vi "DCA Convert Measurement Cluster.vi"(4 "Conversion":enum16{"Cluster - HTML", "HTML - Cluster"}(ring), 6 "Measurements Key Array In":T4, 7 "Measurements Cluster In":T1={"Topology"=enum."PI-Network", "Lock Topology"=FALSE, "ATTN Calc"=enum."Power", "Zo"=50.0}) -> (1 "Measurements Cluster Out":T1={"Topology"=enum."PI-Network", "Lock Topology"=FALSE, "ATTN Calc"=enum."Power", "Zo"=50.0}, 2 "Measurements HTML Out":string)   [LabVIEW 2011]
uses:
  Addons/internet/utils/keyedarr.llb/Keyed Array.ctl
  TypeDefs/DCA Measurement Cluster.ctl
  TypeDefs/DCA Topology.ctl
  TypeDefs/DCA Attenuation Calculation.ctl
  Addons/internet/utils/strutil.llb/Case Matching.ctl
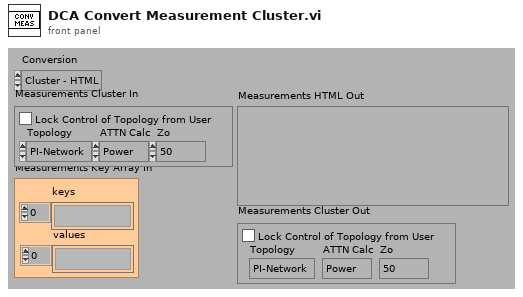
[diagram p1: front panel]
types:
  T1 = typedef "DCA Measurement Cluster.ctl" = cluster{"Topology":T2, "Lock Topology":bool, "ATTN Calc":T3, "Zo":dbl}
  T2 = typedef "DCA Topology.ctl" = enum32{"PI-Network", "T-Network"}
  T3 = typedef "DCA Attenuation Calculation.ctl" = enum32{"Power", "Voltage"}
  T4 = typedef "Keyed Array.ctl" = cluster{"keys":string[], "values":string[]}
  T5 = typedef "Case Matching.ctl" = enum16{"a != A", "a == A", "system"}
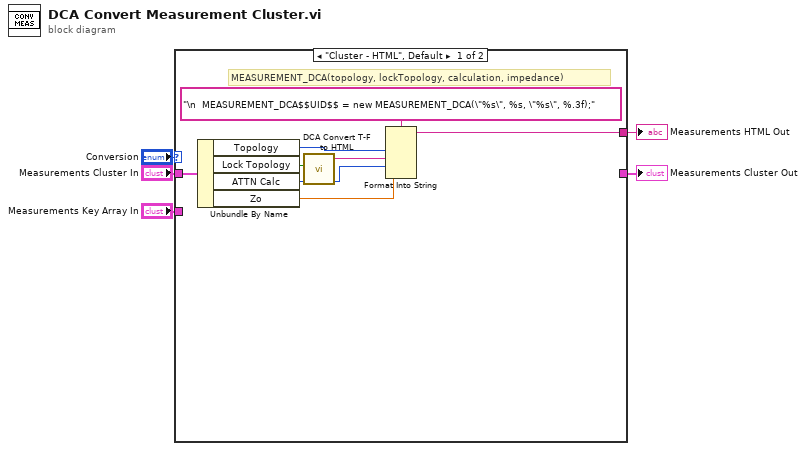
[diagram p0: block diagram]
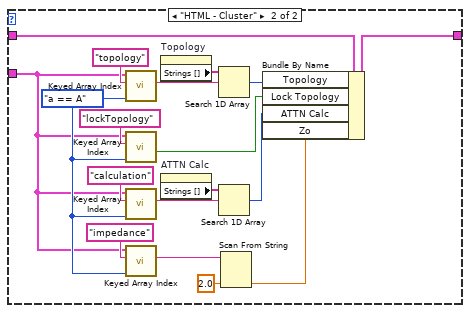
[diagram p2: hidden frame]
diagram:
  n1 = case shown="\"Cluster - HTML\", Default" "Conversion" {
    tunnel: "Measurements Cluster In" -> [w13 w28]
    tunnel: "Measurements Key Array In" -> [_ w20]
    tunnel: [w11 _] -> w2
    tunnel: [_ w27] -> w1
    frame "Cluster - HTML", Default {
      # "MEASUREMENT_DCA(topology, lockTopology, calculation, impedance)"
      n2 = Unbundle By Name(w13) -> ("Topology"=w10:T2, "Lock Topology"=w9:bool, "ATTN Calc"=w7:T3, "Zo"=w6:dbl)
      n3 = call "DCA Convert T-F to HTML.vi"("(T/F)"=w9) -> ("HTML (true/false)"=w8:string)  [unwired: 10 out]
      n4 = Format Into String(format string="\n  MEASUREMENT_DCA$$UID$$ = new MEASUREMENT_DCA(\"%s\", %s, \"%s\", %.3f);", w10, w8, w7, w6) -> (resulting string=w11:string)  [unwired: 2 in, 1 out]
    }
    frame "HTML - Cluster" {
      w21 = Case_Matching."a == A" ("case matching (sensitive)")
      n5 = call "Keyed Array Index.vi"("case matching (sensitive)"=w21, "key"="topology", "array in"=w20) -> ("value"=w23:string)  [unwired: 1 in, 3 out]
      n6 = call "Keyed Array Index.vi"("case matching (sensitive)"=w21, "key"="lockTopology", "array in"=w20) -> ("valid key"=w19:bool)  [unwired: 1 in, 3 out]
      n7 = call "Keyed Array Index.vi"("case matching (sensitive)"=w21, "key"="calculation", "array in"=w20) -> ("value"=w16:string)  [unwired: 1 in, 3 out]
      n8 = call "Keyed Array Index.vi"("case matching (sensitive)"=w21, "key"="impedance", "array in"=w20) -> ("value"=w18:string)  [unwired: 1 in, 3 out]
      n9 = property on="Topology" class="Enum (strict)"() -> ("Strings []"=w24:string[])  [unwired: 2 in, 2 out]
      n10 = property on="ATTN Calc" class="Enum (strict)"() -> ("Strings []"=w17:string[])  [unwired: 2 in, 2 out]
      n11 = Search 1D Array(1D array=w24, element=w23) -> (index of element=w22:i32)  [unwired: 1 out]
      n12 = Search 1D Array(1D array=w17, element=w16) -> (index of element=w15:i32)  [unwired: 1 out]
      n13 = Scan From String(input string=w18, default 1=2.0 ("default value 1")) -> (output 1=w14:dbl)  [unwired: 3 in, 3 out]
      n14 = Bundle By Name(cluster=w28, "Topology"=w22, "Lock Topology"=w19, "ATTN Calc"=w15, "Zo"=w14) -> (w27:T1)
    }
  }
  "Measurements HTML Out" <- w2
  "Measurements Cluster Out" <- w1
